vi "Testbench ZBX IO Arbiter.vi"() -> ()   [LabVIEW 2023]
uses:
  <vilib>/Analysis/NI_AALBase.lvlib
  <instrlib>/niUSRP/Reference FPGA/ZBX Control/ZBX IO Response.ctl
  <instrlib>/_niInstr/Basic Elements/v1/FPGA/Private/Count Down U64.vi
panel:
  out "iterations":i32
  out "message":string
  out "requests order correct":bool
  out "requests data correct":bool
  out "request read or write is always a 1 cycle pulse":bool
  out "Requests input vs. output":cluster{u16[]}[](graph)
  out "collisions":i16
  out "Timeline requests/collisions/response time":cluster{i16[]}[](graph)
  out "pass":bool
  out "protocol violations":u64
  in  "max wait time between requests [cycles]":i32=25
  in  "#requests 2":u16=1000
  out "seed":i32=1
  in  "#requests 1":u16=1000
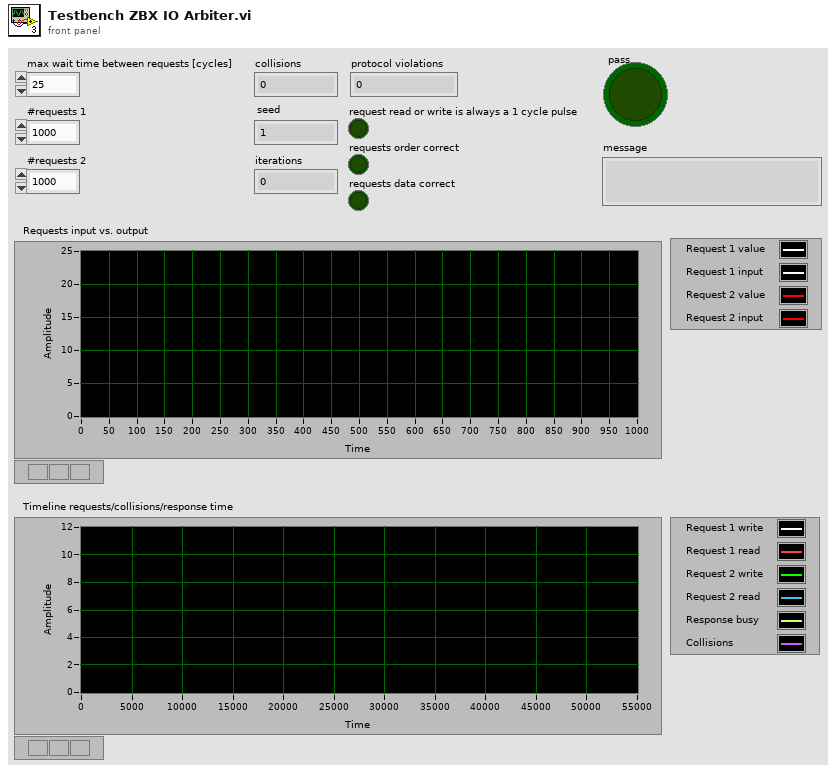
[diagram p1: front panel]
types:
  T1 = typedef "ZBX IO Response.ctl" = cluster{"response Ack":bool, "response data":u32, "response status":fxp<+,2,2>}
  T2 = typedef "ZBX IO Request.ctl" = cluster{"I/O Address":fxp<+,20,20>, "I/O Request Data":u32, "request write":bool, "request read":bool, "request has time":bool, "request time":u64}
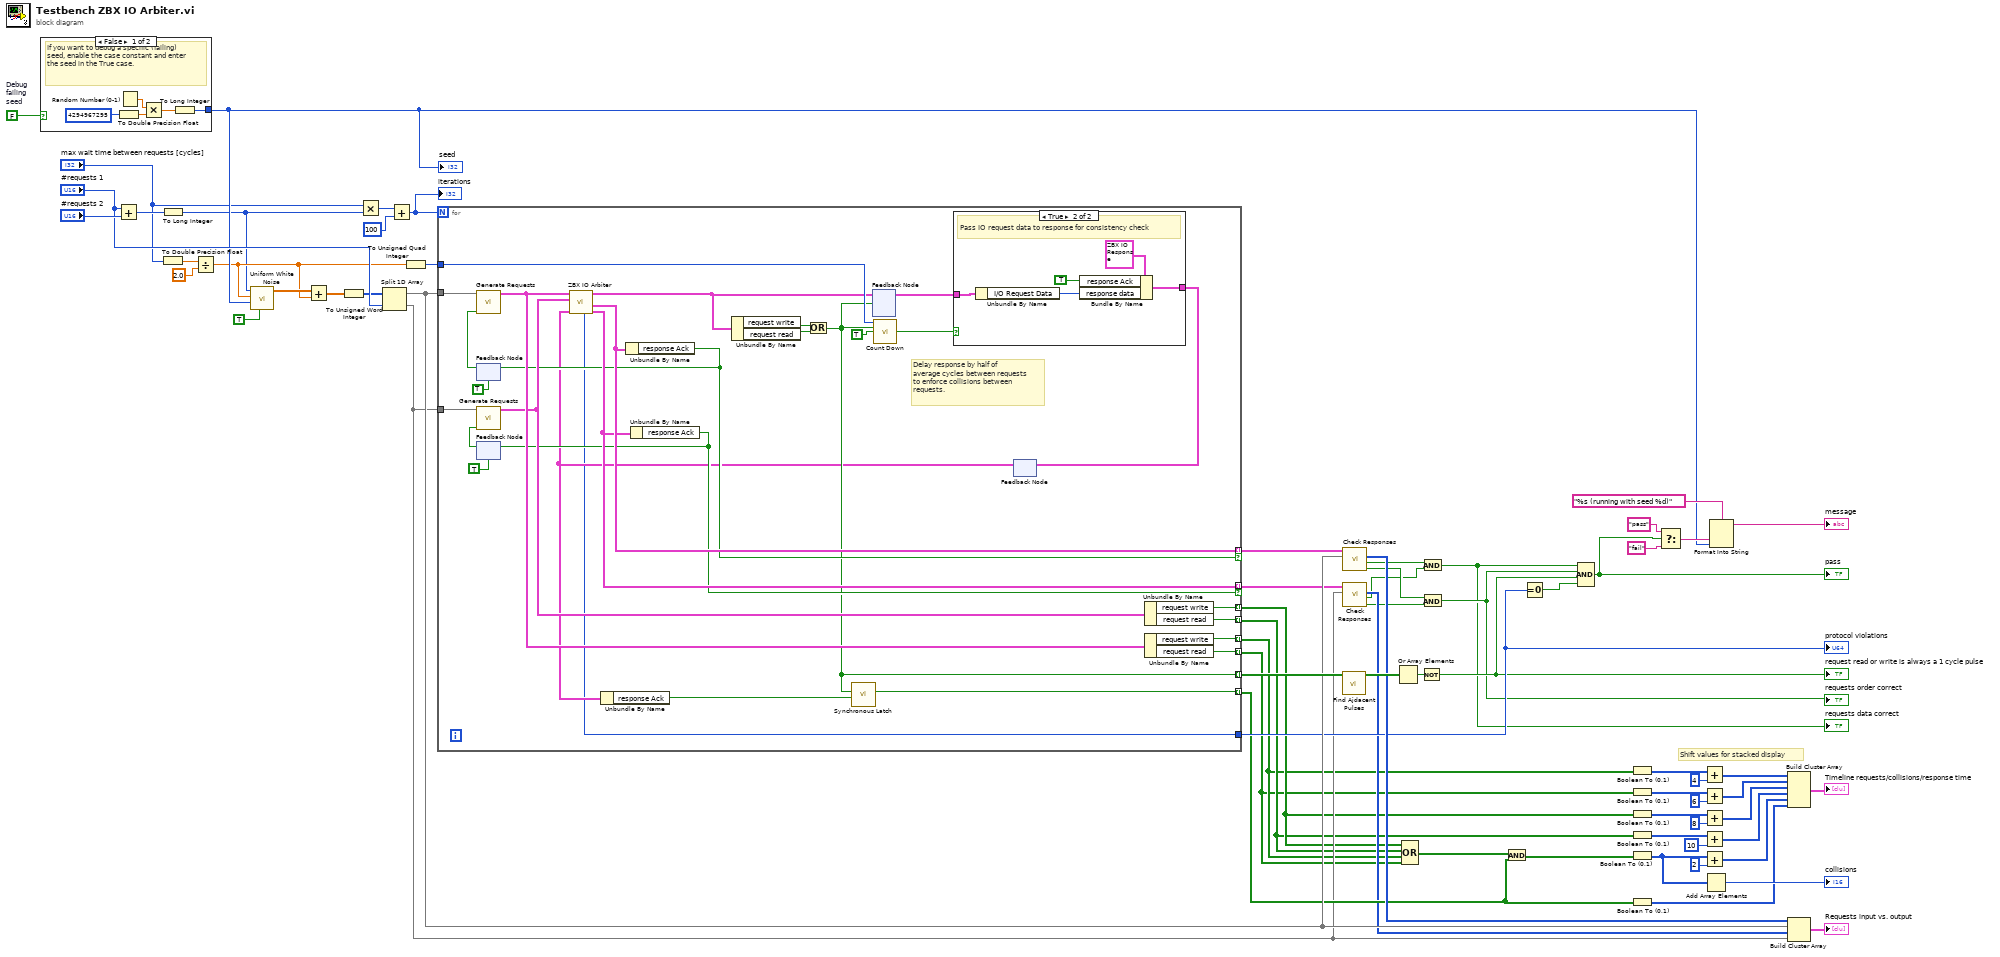
[diagram p0: block diagram]
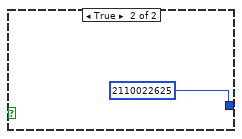
[diagram p3: hidden frame]
diagram:
  w23 = FALSE  # Debug failing seed
  # "Shift values for stacked display"
  n1 = case shown="False" w23 {
    tunnel: [w71 2110022625 ("32bit integer")] -> w24
    frame False {
      # "If you want to debug a specific (failing) seed, enable the case constant and enter the seed in the True case."
      n2 = To Double Precision Float(number=u32 4294967295) -> (double precision float=w69:dbl)
      n3 = Random Number (0-1)() -> (number: 0 to 1=w73:dbl)
      n4 = Multiply(x=w73, y=w69) -> (x*y=w72:dbl)
      n5 = To Long Integer(number=w72) -> (32bit integer=w71:i32)
    }
    frame True {
    }
  }
  "seed" <- w24
  n6 = Add(x="#requests 1", y="#requests 2") -> (x+y=w19:u16)
  n7 = To Long Integer(number=w19) -> (32bit integer=w5:i32)
  n8 = To Double Precision Float(number="max wait time between requests [cycles]") -> (double precision float=w26:dbl)
  n9 = Divide(x=w26, y=2.0) -> (x/y=w22:dbl)
  n10 = call <vilib>:"Uniform White Noise.vi"("initialize?"=TRUE, "seed"=w24, "amplitude"=w22, "samples"=w5) -> ("uniform white noise"=w67:dbl[])  [unwired: 6 in, 1 out]
  n11 = Add(x=w67, y=w22) -> (x+y=w41:dbl[])
  n12 = To Unsigned Word Integer(number=w41) -> (unsigned 16bit integer=w42:u16[])
  n13 = Multiply(x="max wait time between requests [cycles]", y=w5) -> (x*y=w17:i32)
  n14 = Split 1D Array(array=w42, index="#requests 1") -> (first subarray=w38:u16[], second subarray=w14:u16[])
  n15 = Add(x=w17, y=100) -> (x+y=w6:i32)
  "iterations" <- w6
  n16 = To Unsigned Quad Integer(1:w22) -> (0:w21:u64)
  n17 = for {
    N: w6 -> [_]
    tunnel: w38 -> [w103]
    tunnel: w14 -> [w102]
    tunnel: [w98] -> w8 mode=indexing
    tunnel: [w97] -> w9 mode=indexing
    tunnel: [w96] -> w7 mode=indexing
    tunnel: [w95] -> w10 mode=indexing
    tunnel: [w91] -> w64 mode=indexing if=w89
    tunnel: [w81] -> w62 mode=indexing
    tunnel: [w90] -> w15 mode=indexing if=w87
    tunnel: [w77] -> w37
    tunnel: w21 -> [w85]
    tunnel: [w78] -> w20 mode=indexing
    # "Delay response by half of\naverage cycles between requests\nto enforce collisions between\nrequests."
    n18 = feedback #1(TRUE ("response Ack")) -> (w75:bool)
    n19 = call <instrlib>:"Generate Requests.vi"("trigger"=w75, "delays"=w103) -> ("request"=w100:T2)  [unwired: 9 in]
    n20 = feedback #2(TRUE ("terminal count")) -> (w76:bool)
    n21 = call <instrlib>:"Generate Requests.vi"("trigger"=w76, "delays"=w102) -> ("request"=w99:T2)  [unwired: 9 in]
    n22 = feedback #3() -> (w82:T2)  [unwired: 1 in]
    n23 = feedback #4() -> (w80:T1)  [unwired: 1 in]
    n24 = call <instrlib>:"ZBX IO Arbiter.vi"("response"=w80, "request 2"=w99, "request 1"=w100) -> ("response 2"=w90:T1, "response1"=w91:T1, "request out"=w83:T2, "protocol violation"=w77:u64)  [unwired: 5 in]
    n25 = Unbundle By Name(w80) -> ("response Ack"=w79:bool)
    n26 = Unbundle By Name(w91) -> ("response Ack"=w89:bool)
    n27 = feedback-in #1(w89) -> ()
    n28 = Unbundle By Name(w90) -> ("response Ack"=w87:bool)
    n29 = feedback-in #2(w87) -> ()
    n30 = Unbundle By Name(w83) -> ("request write"=w94:bool, "request read"=w93:bool)
    n31 = Or(x=w94, y=w93) -> (x .or. y?=w81:bool)
    n32 = call <instrlib>:"Synchronous Latch.vi"("clear"=w79, "set"=w81) -> ("out"=w78:bool)  [unwired: 9 in]
    n33 = feedback-in #3(w83, w81) -> ()
    n34 = call-poly <instrlib>:"Count Down.vi"("count in"=w85, "load"=w81, "decrement"=TRUE) -> ("terminal count"=w84:bool)  [unwired: 11 in, 1 out]
    n35 = case shown="True" w84 {
      tunnel: w82 -> [_ w108]
      tunnel: [_ w105] -> w92
      frame False {
      }
      frame True {
        # "Pass IO request data to response for consistency check"
        n36 = Unbundle By Name(w108) -> ("I/O Request Data"=w106:u32)
        n37 = Bundle By Name(cluster=T1 {"response Ack"=FALSE, "response data"=0, "response status"=0.0} ("response"), "response Ack"=TRUE, "response data"=w106) -> (w105:T1)
      }
    }
    n38 = feedback-in #4(w92) -> ()
    n39 = Unbundle By Name(w99) -> ("request write"=w95:bool, "request read"=w97:bool)
    n40 = Unbundle By Name(w100) -> ("request write"=w98:bool, "request read"=w96:bool)
  }
  "protocol violations" <- w37
  n41 = call <instrlib>:"Find Ajdacent Pulses.vi"("Array in"=w62) -> ("Array out"=w63:bool[])  [unwired: 10 in]
  n42 = call <instrlib>:"Check Responses.vi"("delays"=w38, "responses"=w64) -> ("consecutive requests?"=w3:bool, "delays match?"=w2:bool, "response delays"=w40:u16[])  [unwired: 7 in]
  n43 = call <instrlib>:"Check Responses.vi"("delays"=w14, "responses"=w15) -> ("consecutive requests?"=w4:bool, "delays match?"=w1:bool, "response delays"=w13:u16[])  [unwired: 7 in]
  n44 = Or Array Elements(Boolean array=w63) -> (logical OR=w35:bool)
  n45 = Compound Arithmetic op=OR(w10, w9, w8, w7) -> (w49:bool[])
  n46 = Not(x=w35) -> (.not. x?=w34:bool)
  "request read or write is always a 1 cycle pulse" <- w34
  n47 = And(x=w2, y=w1) -> (x .and. y?=w12:bool)
  "requests data correct" <- w12
  n48 = And(x=w3, y=w4) -> (x .and. y?=w33:bool)
  "requests order correct" <- w33
  n49 = And(x=w49, y=w20) -> (x .and. y?=w48:bool[])
  n50 = Equal To 0?(x=w37) -> (x = 0?=w36:bool)
  n51 = Compound Arithmetic op=AND(w12, w33, w34, w36) -> (w30:bool)
  "pass" <- w30
  n52 = Boolean To (0,1)(Boolean=w8) -> (0, 1=w52:i16[])
  n53 = Boolean To (0,1)(Boolean=w7) -> (0, 1=w59:i16[])
  n54 = Boolean To (0,1)(Boolean=w10) -> (0, 1=w56:i16[])
  n55 = Boolean To (0,1)(Boolean=w9) -> (0, 1=w54:i16[])
  n56 = Boolean To (0,1)(Boolean=w48) -> (0, 1=w46:i16[])
  n57 = Boolean To (0,1)(Boolean=w20) -> (0, 1=w43:i16[])
  n58 = Select(t="pass" ("format string"), s=w30, f="fail") -> (s? t:f=w27:string)
  n59 = Add(x=w52, y=i16 4) -> (x+y=w51:i16[])
  n60 = Add(x=w59, y=i16 6) -> (x+y=w58:i16[])
  n61 = Add(x=w56, y=i16 8) -> (x+y=w55:i16[])
  n62 = Add(x=w54, y=i16 10) -> (x+y=w11:i16[])
  n63 = Add(x=w46, y=i16 2) -> (x+y=w44:i16[])
  n64 = Add Array Elements(numeric array=w46) -> (sum=→"collisions":i16)
  n65 = Format Into String(format string="%s (running with seed %d)", w27, w24) -> (resulting string=→"message":string)  [unwired: 2 in, 1 out]
  n66 = Build Cluster Array(w51, w58, w55, w11, w44, w43) -> (→"Timeline requests/collisions/response time":cluster{i16[]}[])
  n67 = Build Cluster Array(w40, w38, w13, w14) -> (→"Requests input vs. output":cluster{"response delays":u16[]}[])
